vi "Assert Floating Point wired to Int Type.vi"   [LabVIEW 2017]
uses:
  455eed85-9c29-4121-af11-d9cb0bec3e29.vi
  b044ac8e-82c3-4b9a-a16b-66d0f1074277.vi
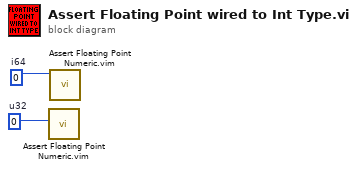
[diagram p0: block diagram]
diagram:
  w1 = u32 0  # u32
  w2 = i64 0  # i64
  n1 = call "Assert Floating Point Numeric.vim"("Input"=w1) -> ()  [unwired: 10 in, 1 out]
  n2 = call "Assert Floating Point Numeric.vim"("Input"=w2) -> ()  [unwired: 10 in, 1 out]
